vi "Omniax_mDrive_COM9.vi"() -> ()   [LabVIEW 2009]
uses:
  <vilib>/Instr/_visa.llb/VISA Configure Serial Port (Instr).vi
panel:
  out "Holding Current %":i32
  out "Run Current %":i32
  out "slew velocity mm/sec":dbl
  out "slew length mm":dbl
  in  "Slew Cancel":bool
  out "Position mm":dbl
  out "offset":dbl
  out "mm/rev":dbl
  out "step/rev":u32
  out "steps/sec":i32
  in  "Slew Length":i32 min=-80000 max=2000 step=100
  out "Slew Ready":bool
  in  "Slew Set":bool
  in  "Slew Go":bool
  in  "Velocity":i32 caption="steps/sec"
  in  "Slew Velocity":i32 min=1 max=1 step=1
  in  "Backlash":i32
  in  "Stop":bool
  out "In Range?":bool
  out "Current Values":i32 max=2000
  out "Status":string
  in  "Go":bool
  in  "Move to":i32=-20000 min=-80000 max=2000 step=500
  out "MINPOS":i32=-94296
  out "MAXPOS":i32=-34296
  out "COM PORT":refnum<visa-resource-name>="COM5"
  # "SY"
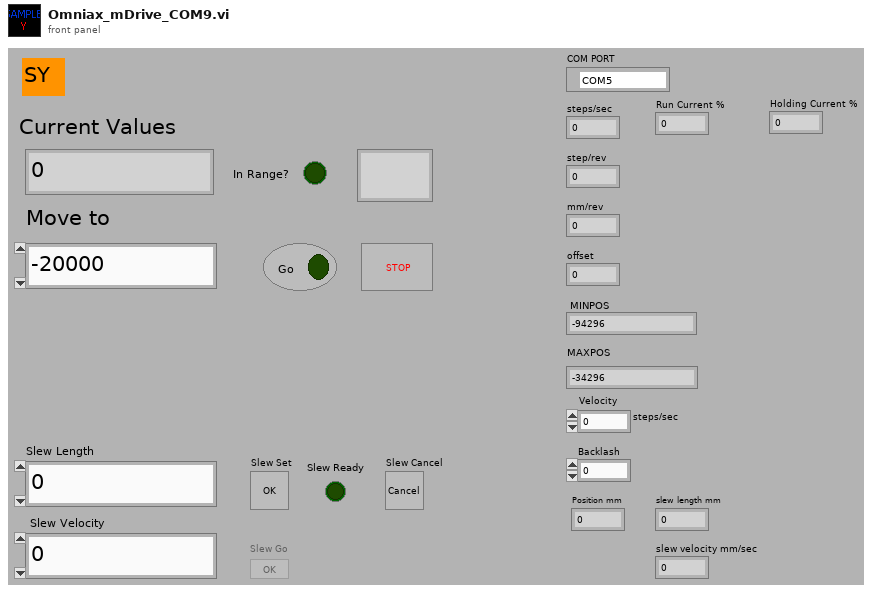
[diagram p1: front panel]
types:
  T1 = enum8{"Enabled", "Disabled", "Disabled and Grayed Out"}
  T2 = enum16{"Stop", "Reset", "Run Current", "Holding Current", "Accel Rate", "Decel Rate", "Move to Relative Position", "Move to Absolute Position", "Prtint Position", "Print Encorder", "Print Velocity Maximum", "Print Velocity", "Microstep Resolution", "Hold", "Max Velocity"}
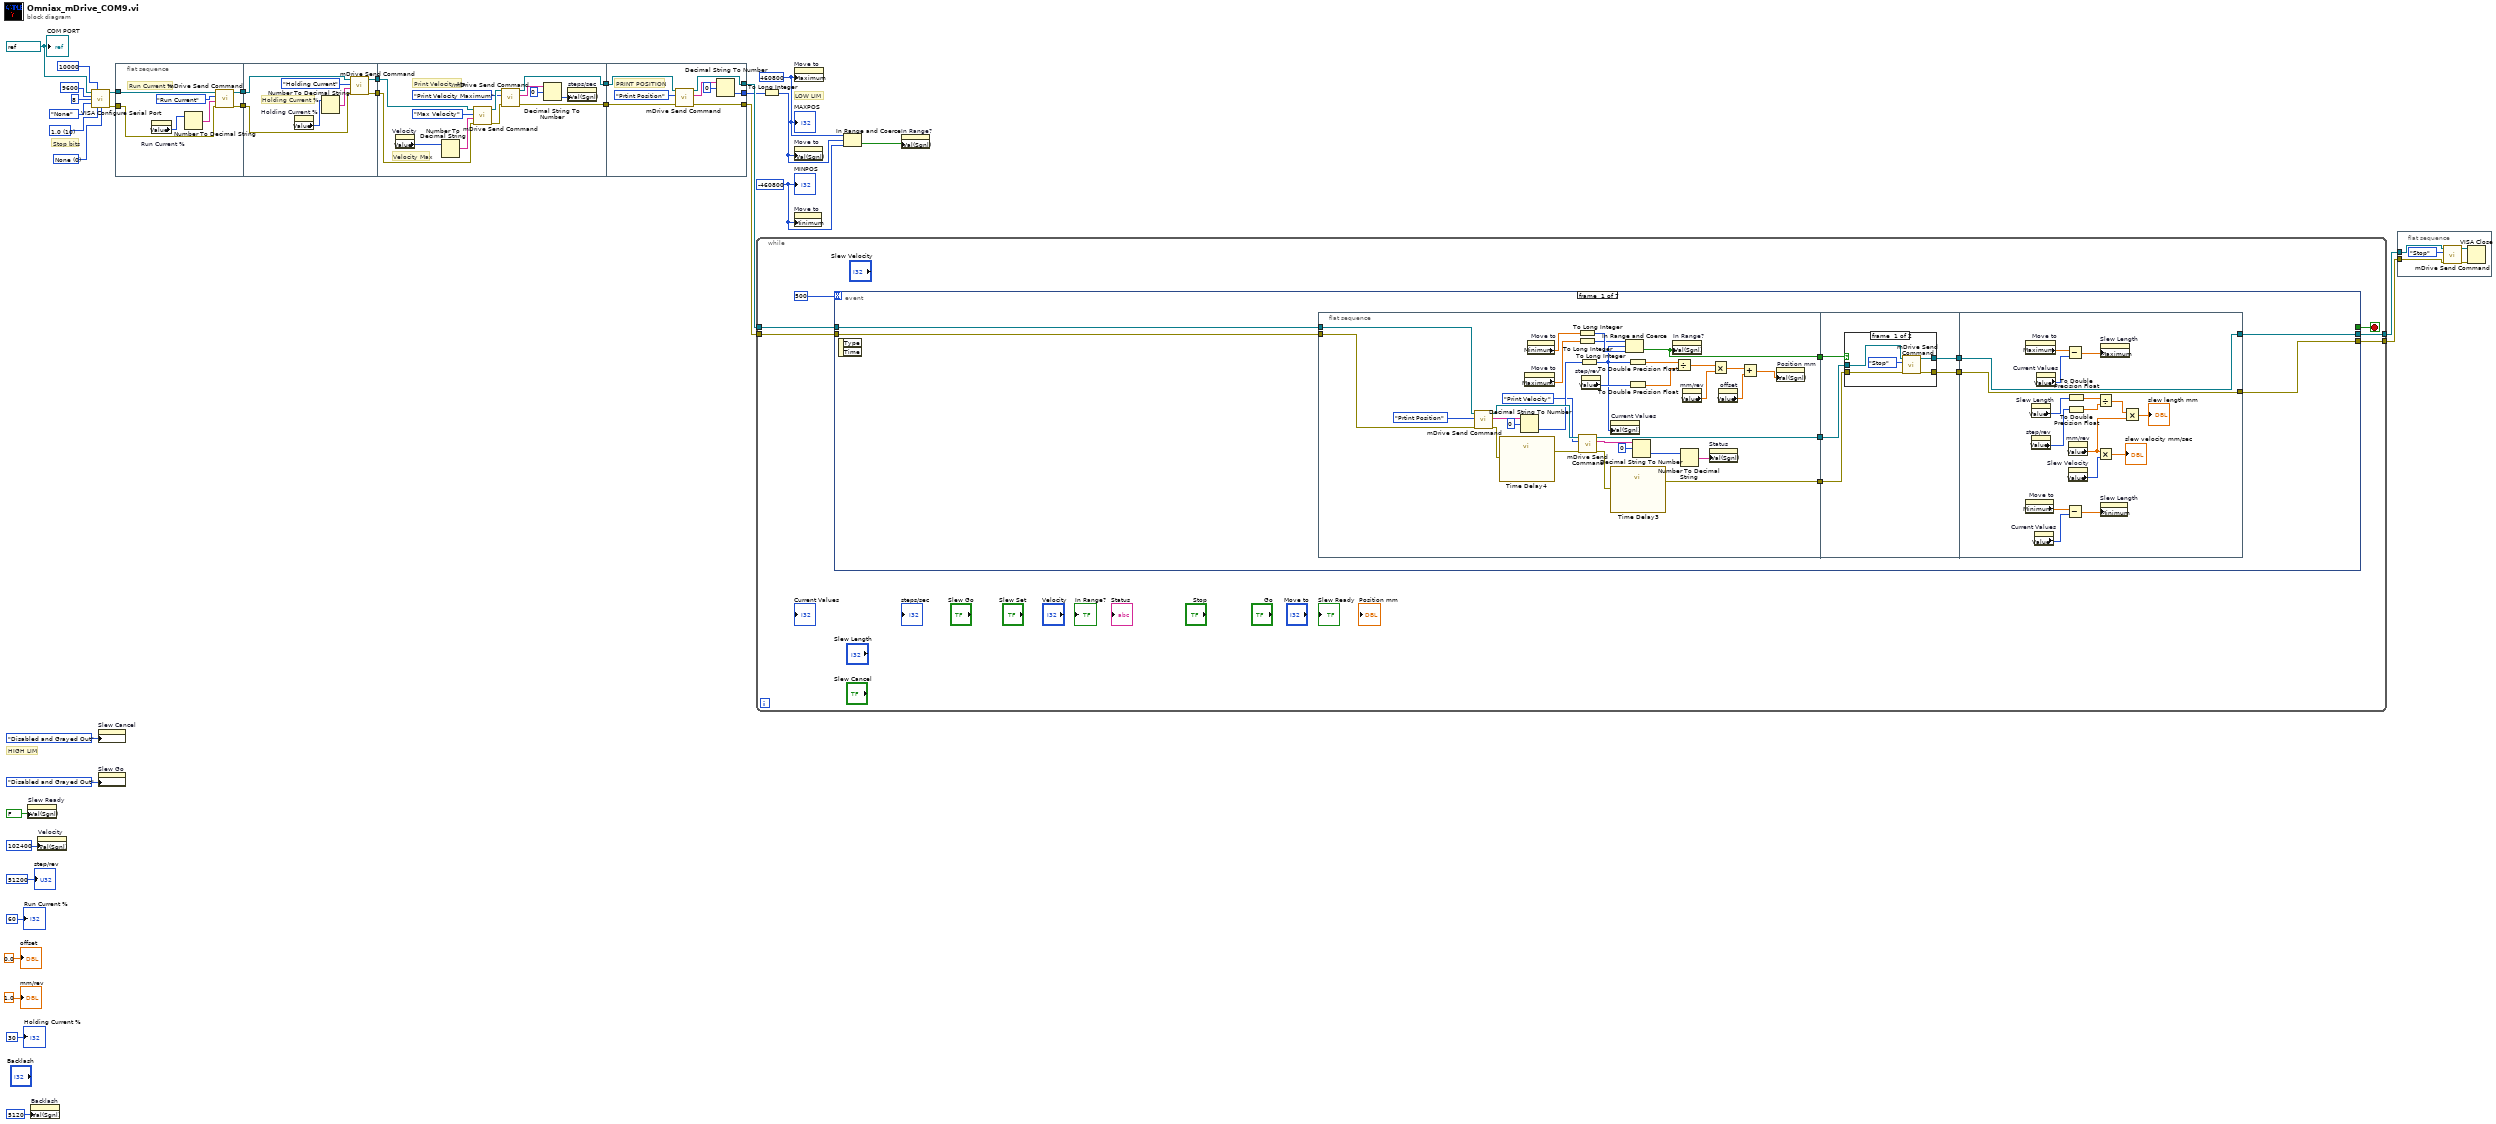
[diagram p0: block diagram]
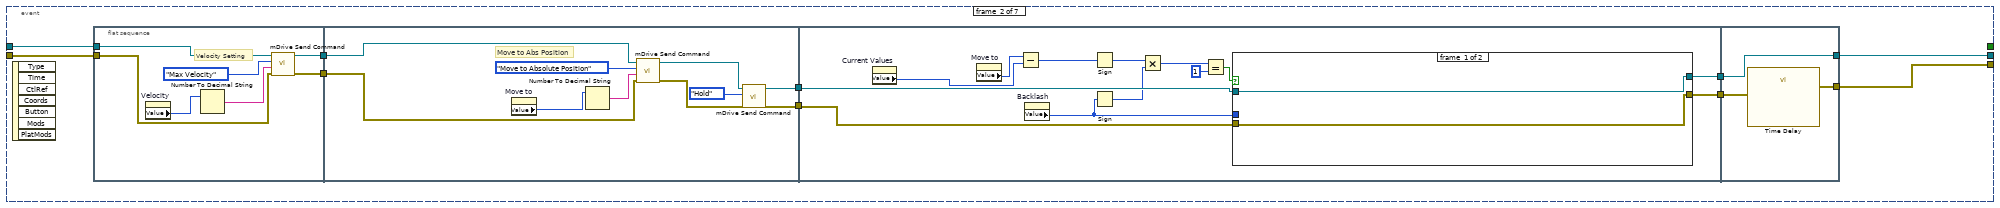
[diagram p3: hidden frame]
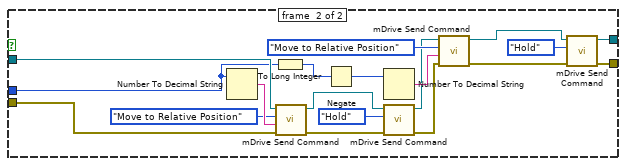
[diagram p4: hidden frame]
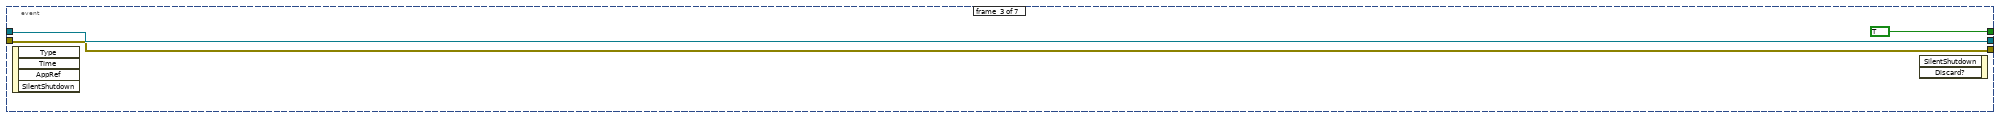
[diagram p5: hidden frame]
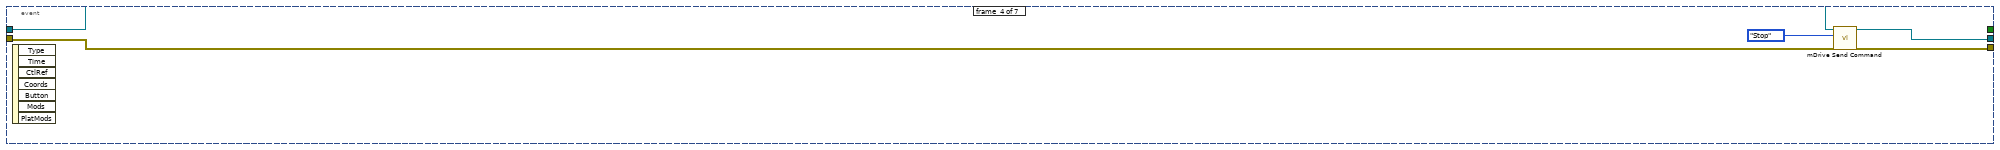
[diagram p6: hidden frame]
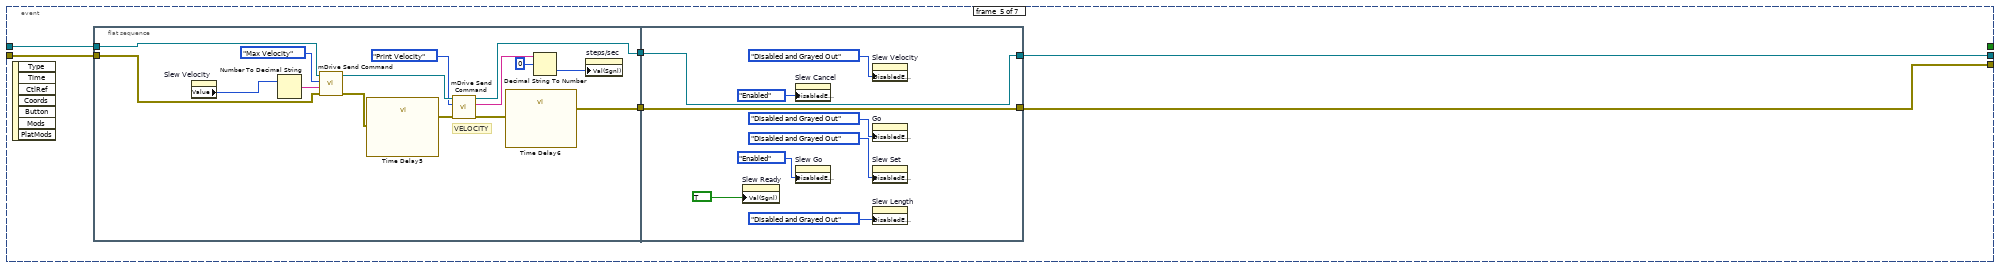
[diagram p7: hidden frame]
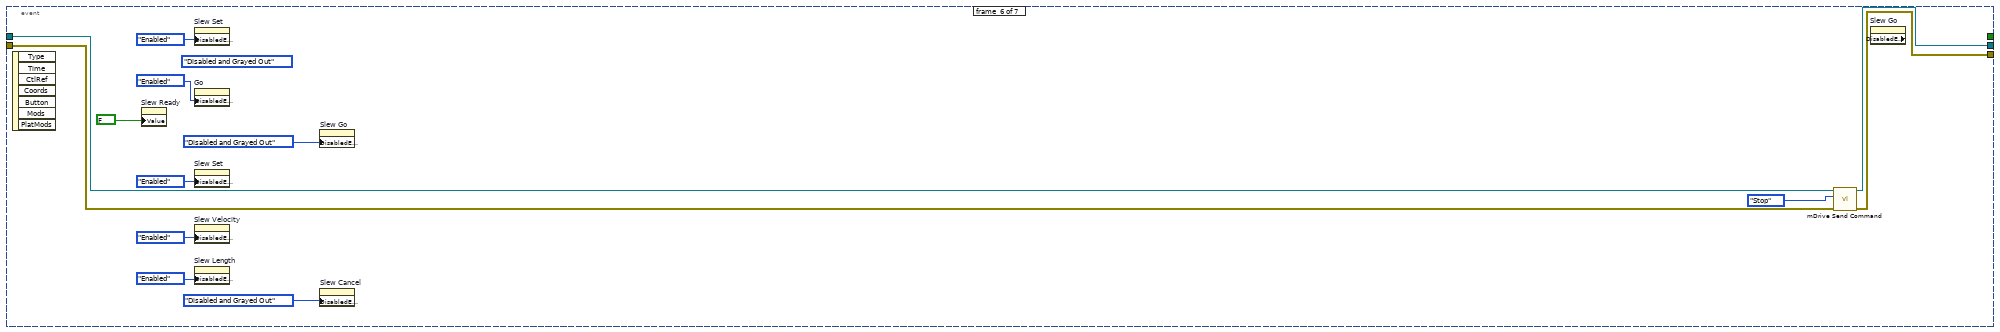
[diagram p8: hidden frame]
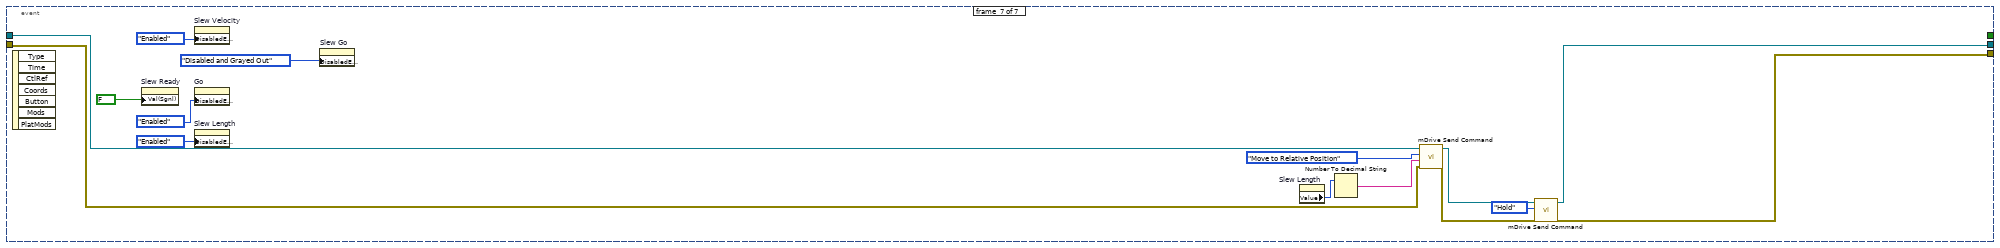
[diagram p9: hidden frame]
diagram:
  w20 = -460800 ("lower limit")
  w19 = 460800 ("upper limit")
  w28 = refnum<visa-resource-name> "COM9" ("COM PORT")
  w30 = u16 0 items=["None", "XON/XOFF", "RTS/CTS", "XON/XOFF & RTS/CTS", "DTR/DSR", "XON/XOFF & DTR/DSR"] ("flow control (0:none)")
  w31 = u16 10 items=["1.0"=10, "1.5"=15, "2.0"=20] ("stop bits (10: 1 bit)")
  # "HIGH LIM"
  # "LOW LIM"
  # "Stop bits"
  n1 = property on="Slew Ready" class="Bool (strict)"("Val(Sgnl)"=FALSE ("Value (Signaling)")) -> ()  [unwired: 2 in, 2 out]
  n2 = property on="Backlash" class="DigNum (strict)"("Val(Sgnl)"=u32 5120 ("Value (Signaling)")) -> ()  [unwired: 2 in, 2 out]
  n3 = property on="Velocity" class="DigNum (strict)"("Val(Sgnl)"=102400 ("Value (Signaling)")) -> ()  [unwired: 2 in, 2 out]
  n4 = call-poly "VISA Configure Serial Port"("VISA resource name"=w28, "timeout (10sec)"=u32 10000, "baud rate (9600)"=u32 9600, "data bits (8)"=u16 8, "parity (0:none)"=enum16{"None", "Odd", "Even", "Mark", "Space"}."None", "stop bits (10: 1 bit)"=w31, "flow control (0:none)"=w30) -> ("VISA resource name out"=w14:refnum<visa-resource-name>, "error out"=w13:errorcluster)  [unwired: 7 in]
  n5 = property on="Slew Cancel" class="Bool"("DisabledEnum"=T1."Disabled and Grayed Out" ("Disabled")) -> ()  [unwired: 2 in, 2 out]
  n6 = property on="Slew Go" class="Bool"("DisabledEnum"=T1."Disabled and Grayed Out" ("Disabled")) -> ()  [unwired: 2 in, 2 out]
  n7 = flat-sequence {
    tunnel: w13 -> [w41]
    tunnel: w14 -> [w39]
    tunnel: [w38] -> w6
    tunnel: [w40] -> w4
    tunnel: w6 -> [w48]
    tunnel: [w47] -> w5
    tunnel: w4 -> [w45]
    tunnel: [w46] -> w3
    tunnel: [w57] -> w16
    tunnel: [w58] -> w15
    tunnel: w5 -> [w56]
    tunnel: w3 -> [w55]
    tunnel: [w69] -> w27
    tunnel: [w68] -> w26
    tunnel: [w63] -> w17
    tunnel: w16 -> [w67]
    tunnel: w15 -> [w66]
    frame #0 {
      # "Run Current %"
      n8 = property on="Run Current %" class="DigNum (strict)"() -> ("Value"=w36:i32)  [unwired: 2 in, 2 out]
      n9 = Number To Decimal String(number=w36) -> (decimal integer string=w37:string)  [unwired: 1 in]
      n10 = call "mDrive Send Command.vi"("error in (no error)"=w41, "Extra"=w37, "Command"=T2."Run Current", "VISA resource name"=w39) -> ("error out"=w40:errorcluster, "VISA resource name out"=w38:refnum<visa-resource-name>)  [unwired: 3 in, 1 out]
    }
    frame #1 {
      # "Holding Current %"
      n11 = property on="Holding Current %" class="DigNum (strict)"() -> ("Value"=w43:i32)  [unwired: 2 in, 2 out]
      n12 = Number To Decimal String(number=w43) -> (decimal integer string=w44:string)  [unwired: 1 in]
      n13 = call "mDrive Send Command.vi"("error in (no error)"=w45, "Extra"=w44, "Command"=T2."Holding Current", "VISA resource name"=w48) -> ("error out"=w46:errorcluster, "VISA resource name out"=w47:refnum<visa-resource-name>)  [unwired: 3 in, 1 out]
    }
    frame #2 {
      # "Print Velocity Ma"
      # "Velocity Max"
      n14 = property on="Velocity" class="DigNum (strict)"() -> ("Value"=w54:i32)  [unwired: 2 in, 2 out]
      n15 = Number To Decimal String(number=w54) -> (decimal integer string=w53:string)  [unwired: 1 in]
      n16 = call "mDrive Send Command.vi"("error in (no error)"=w55, "Extra"=w53, "Command"=T2."Max Velocity", "VISA resource name"=w56) -> ("error out"=w51:errorcluster, "VISA resource name out"=w61:refnum<visa-resource-name>)  [unwired: 3 in, 1 out]
      n17 = call "mDrive Send Command.vi"("error in (no error)"=w51, "Command"=T2."Print Velocity Maximum", "VISA resource name"=w61) -> ("error out"=w58:errorcluster, "read buffer"=w59:string, "VISA resource name out"=w57:refnum<visa-resource-name>)  [unwired: 4 in]
      n18 = Decimal String To Number(string=w59, offset=0) -> (number=w52:i32)  [unwired: 1 in, 1 out]
      n19 = property on="steps/sec" class="DigNum (strict)"("Val(Sgnl)"=w52) -> ()  [unwired: 2 in, 2 out]
    }
    frame #3 {
      # "PRINT POSITION"
      n20 = call "mDrive Send Command.vi"("error in (no error)"=w66, "Command"=T2."Prtint Position", "VISA resource name"=w67) -> ("error out"=w68:errorcluster, "read buffer"=w65:string, "VISA resource name out"=w69:refnum<visa-resource-name>)  [unwired: 4 in]
      n21 = Decimal String To Number(string=w65, offset=0) -> (number=w63:i32)  [unwired: 1 in, 1 out]
    }
  }
  n22 = while {
    tunnel: w27 -> [w71]
    tunnel: w26 -> [w74]
    tunnel: [w75] -> w23
    tunnel: [w73] -> w24
    stop <- w70 stop-if-true
    n23 = event shown="[6] \"Slew Go\": Mouse Up" {
      selector: _ -> [_ _ _ _ _ _ _]
      dyn-events: _ -> [_ _ _ _ _ _ _]
      timeout: 500 -> [_ _ _ _ _ _ _]
      tunnel: w74 -> [w84 w154 w210 w215 w222 w252 w267]
      tunnel: [w83 w151 w210 w213 w220 w254 w261] -> w75
      tunnel: w71 -> [w81 w153 w211 w216 w221 w253 w266]
      tunnel: [w82 w152 w211 w214 w217 w255 w263] -> w73
      tunnel: [_ _ TRUE _ _ _ _] -> w70
      event #0 {
        n24 = event-data() -> ()  [unwired: 1 in, 2 out]
        n25 = flat-sequence {
          tunnel: w84 -> [w110]
          tunnel: w81 -> [w109]
          tunnel: [w115] -> w80
          tunnel: [w89] -> w78
          tunnel: [w102] -> w76
          tunnel: w80 -> [w117]
          tunnel: [w118] -> w79
          tunnel: w78 -> [w120]
          tunnel: [w119] -> w77
          tunnel: w76 -> [w116]
          tunnel: [w143] -> w83
          tunnel: [w144] -> w82
          tunnel: w79 -> [w144]
          tunnel: w77 -> [w143]
          frame #0 {
            n26 = call "mDrive Send Command.vi"("error in (no error)"=w110, "Command"=T2."Prtint Position", "VISA resource name"=w109) -> ("error out"=w108:errorcluster, "read buffer"=w114:string, "VISA resource name out"=w112:refnum<visa-resource-name>)  [unwired: 4 in]
            n27 = call "Time Delay4"("error in (no error)"=w108) -> ("error out"=w107:errorcluster)  [unwired: 10 in]
            n28 = Decimal String To Number(string=w114, offset=0) -> (number=w92:i32)  [unwired: 1 in, 1 out]
            n29 = property on="Move to" class="DigNum (strict)"() -> ("Maximum"=w104:dbl)  [unwired: 2 in, 2 out]
            n30 = property on="Move to" class="DigNum (strict)"() -> ("Minimum"=w106:dbl)  [unwired: 2 in, 2 out]
            n31 = To Long Integer(number=w106) -> (32bit integer=w105:i32)
            n32 = To Long Integer(number=w104) -> (32bit integer=w103:i32)
            n33 = call "mDrive Send Command.vi"("error in (no error)"=w107, "Command"=T2."Print Velocity", "VISA resource name"=w112) -> ("error out"=w111:errorcluster, "read buffer"=w90:string, "VISA resource name out"=w115:refnum<visa-resource-name>)  [unwired: 4 in]
            n34 = To Long Integer(number=w92) -> (32bit integer=w94:i32)
            n35 = property on="step/rev" class="DigNum (strict)"() -> ("Value"=w100:u32)  [unwired: 2 in, 2 out]
            n36 = property on="Current Values" class="DigNum (strict)"("Val(Sgnl)"=w94) -> ()  [unwired: 2 in, 2 out]
            n37 = call "Time Delay3"("error in (no error)"=w111) -> ("error out"=w89:errorcluster)  [unwired: 10 in]
            n38 = In Range and Coerce(upper limit=w103, x=w94, lower limit=w105) -> (In Range?=w102:bool)  [unwired: 1 out]
            n39 = To Double Precision Float(number=w94) -> (double precision float=w95:dbl)
            n40 = To Double Precision Float(number=w100) -> (double precision float=w101:dbl)
            n41 = Decimal String To Number(string=w90, offset=0 ("offset (0)")) -> (number=w88:i32)  [unwired: 1 in, 1 out]
            n42 = property on="In Range?" class="Bool (strict)"("Val(Sgnl)"=w102) -> ()  [unwired: 2 in, 2 out]
            n43 = Divide(x=w95, y=w101) -> (x/y=w99:dbl)
            n44 = Number To Decimal String(number=w88) -> (decimal integer string=w87:string)  [unwired: 1 in]
            n45 = property on="mm/rev" class="DigNum (strict)"() -> ("Value"=w98:dbl)  [unwired: 2 in, 2 out]
            n46 = property on="Status" class="Str"("Val(Sgnl)"=w87) -> ()  [unwired: 2 in, 2 out]
            n47 = Multiply(x=w99, y=w98) -> (x*y=w97:dbl)
            n48 = property on="offset" class="DigNum (strict)"() -> ("Value"=w96:dbl)  [unwired: 2 in, 2 out]
            n49 = Add(x=w97, y=w96) -> (x+y=w93:dbl)
            n50 = property on="Position mm" class="DigNum (strict)"("Val(Sgnl)"=w93) -> ()  [unwired: 2 in, 2 out]
          }
          frame #1 {
            n51 = case shown="False" w116 {
              tunnel: w117 -> [w123 w127]
              tunnel: [w124 w127] -> w118
              tunnel: [w125 w126] -> w119
              tunnel: w120 -> [w122 w126]
              frame #0 {
                n52 = call "mDrive Send Command.vi"("error in (no error)"=w122, "Command"=T2."Stop", "VISA resource name"=w123) -> ("error out"=w125:errorcluster, "VISA resource name out"=w124:refnum<visa-resource-name>)  [unwired: 4 in, 1 out]
              }
              frame #1 {
              }
            }
          }
          frame #2 {
            n53 = property on="Move to" class="DigNum (strict)"() -> ("Maximum"=w138:dbl)  [unwired: 2 in, 2 out]
            n54 = property on="Move to" class="DigNum (strict)"() -> ("Minimum"=w140:dbl)  [unwired: 2 in, 2 out]
            n55 = property on="Slew Length" class="DigNum (strict)"() -> ("Value"=w134:i32)  [unwired: 2 in, 2 out]
            n56 = property on="step/rev" class="DigNum (strict)"() -> ("Value"=w132:u32)  [unwired: 2 in, 2 out]
            n57 = property on="Current Values" class="DigNum (strict)"() -> ("Value"=w142:i32)  [unwired: 2 in, 2 out]
            n58 = property on="Current Values" class="DigNum (strict)"() -> ("Value"=w139:i32)  [unwired: 2 in, 2 out]
            n59 = Subtract(x=w138, y=w139) -> (x-y=w137:dbl)
            n60 = Subtract(x=w140, y=w142) -> (x-y=w141:dbl)
            n61 = To Double Precision Float(number=w134) -> (double precision float=w133:dbl)
            n62 = To Double Precision Float(number=w132) -> (double precision float=w136:dbl)
            n63 = property on="mm/rev" class="DigNum (strict)"() -> ("Value"=w128:dbl)  [unwired: 2 in, 2 out]
            n64 = property on="Slew Velocity" class="DigNum (strict)"() -> ("Value"=w130:i32)  [unwired: 2 in, 2 out]
            n65 = Divide(x=w133, y=w136) -> (x/y=w135:dbl)
            n66 = Multiply(x=w128, y=w130) -> (x*y=→"slew velocity mm/sec":dbl)
            n67 = property on="Slew Length" class="DigNum (strict)"("Maximum"=w137) -> ()  [unwired: 2 in, 2 out]
            n68 = property on="Slew Length" class="DigNum (strict)"("Minimum"=w141) -> ()  [unwired: 2 in, 2 out]
            n69 = Multiply(x=w135, y=w128) -> (x*y=→"slew length mm":dbl)
          }
        }
      }
      event #1 {
        n70 = event-data() -> ()  [unwired: 1 in, 7 out]
        n71 = flat-sequence {
          tunnel: w153 -> [w157]
          tunnel: w154 -> [w160]
          tunnel: [w159] -> w147
          tunnel: [w158] -> w146
          tunnel: w147 -> [w170]
          tunnel: w146 -> [w171]
          tunnel: [w165] -> w150
          tunnel: [w163] -> w148
          tunnel: w150 -> [w184]
          tunnel: [w181] -> w149
          tunnel: w148 -> [w183]
          tunnel: [w182] -> w145
          tunnel: [w207] -> w151
          tunnel: [w208] -> w152
          tunnel: w149 -> [w208]
          tunnel: w145 -> [w206]
          frame #0 {
            # "Velocity Setting"
            n72 = property on="Velocity" class="DigNum (strict)"() -> ("Value"=w161:i32)  [unwired: 2 in, 2 out]
            n73 = Number To Decimal String(number=w161) -> (decimal integer string=w156:string)  [unwired: 1 in]
            n74 = call "mDrive Send Command.vi"("error in (no error)"=w160, "Extra"=w156, "Command"=T2."Max Velocity", "VISA resource name"=w157) -> ("error out"=w159:errorcluster, "VISA resource name out"=w158:refnum<visa-resource-name>)  [unwired: 3 in, 1 out]
          }
          frame #1 {
            # "Move to Abs Position"
            n75 = property on="Move to" class="DigNum (strict)"() -> ("Value"=w169:i32)  [unwired: 2 in, 2 out]
            n76 = Number To Decimal String(number=w169) -> (decimal integer string=w168:string)  [unwired: 1 in]
            n77 = call "mDrive Send Command.vi"("error in (no error)"=w170, "Extra"=w168, "Command"=T2."Move to Absolute Position", "VISA resource name"=w171) -> ("error out"=w164:errorcluster, "VISA resource name out"=w166:refnum<visa-resource-name>)  [unwired: 3 in, 1 out]
            n78 = call "mDrive Send Command.vi"("error in (no error)"=w164, "Command"=T2."Hold", "VISA resource name"=w166) -> ("error out"=w163:errorcluster, "VISA resource name out"=w165:refnum<visa-resource-name>)  [unwired: 4 in, 1 out]
          }
          frame #2 {
            n79 = property on="Current Values" class="DigNum (strict)"() -> ("Value"=w179:i32)  [unwired: 2 in, 2 out]
            n80 = property on="Move to" class="DigNum (strict)"() -> ("Value"=w180:i32)  [unwired: 2 in, 2 out]
            n81 = Subtract(x=w180, y=w179) -> (x-y=w178:i32)
            n82 = property on="Backlash" class="DigNum (strict)"() -> ("Value"=w172:i32)  [unwired: 2 in, 2 out]
            n83 = Sign(1:w178) -> (0:w177:i32)
            n84 = Sign(1:w172) -> (0:w176:i32)
            n85 = Multiply(x=w177, y=w176) -> (x*y=w175:i32)
            n86 = Equal?(x=w175, y=1) -> (x = y?=w173:bool)
            n87 = case shown="True" w173 {
              tunnel: w184 -> [w186 w205]
              tunnel: [w186 w187] -> w181
              tunnel: [w185 w189] -> w182
              tunnel: w183 -> [w185 w204]
              tunnel: w172 -> [_ w199]
              frame #0 {
              }
              frame #1 {
                n88 = Number To Decimal String(number=w199) -> (decimal integer string=w203:string)  [unwired: 1 in]
                n89 = To Long Integer(number=w199) -> (32bit integer=w201:i32)
                n90 = call "mDrive Send Command.vi"("error in (no error)"=w204, "Extra"=w203, "Command"=T2."Move to Relative Position", "VISA resource name"=w205) -> ("error out"=w196:errorcluster, "VISA resource name out"=w194:refnum<visa-resource-name>)  [unwired: 3 in, 1 out]
                n91 = Negate(x=w201) -> (-x=w202:i32)
                n92 = Number To Decimal String(number=w202) -> (decimal integer string=w200:string)  [unwired: 1 in]
                n93 = call "mDrive Send Command.vi"("error in (no error)"=w196, "Command"=T2."Hold", "VISA resource name"=w194) -> ("error out"=w195:errorcluster, "VISA resource name out"=w193:refnum<visa-resource-name>)  [unwired: 4 in, 1 out]
                n94 = call "mDrive Send Command.vi"("error in (no error)"=w195, "Extra"=w200, "Command"=T2."Move to Relative Position", "VISA resource name"=w193) -> ("error out"=w190:errorcluster, "VISA resource name out"=w188:refnum<visa-resource-name>)  [unwired: 3 in, 1 out]
                n95 = call "mDrive Send Command.vi"("error in (no error)"=w190, "Command"=T2."Hold", "VISA resource name"=w188) -> ("error out"=w189:errorcluster, "VISA resource name out"=w187:refnum<visa-resource-name>)  [unwired: 4 in, 1 out]
              }
            }
          }
          frame #3 {
            n96 = call "Time Delay"("error in (no error)"=w206) -> ("error out"=w207:errorcluster)  [unwired: 10 in]
          }
        }
      }
      event #2 {
        n97 = event-data() -> ()  [unwired: 1 in, 4 out]
        n98 = event-data() -> ()  [unwired: 3 in, 1 out]
      }
      event #3 {
        n99 = event-data() -> ()  [unwired: 1 in, 7 out]
        n100 = call "mDrive Send Command.vi"("error in (no error)"=w215, "Command"=T2."Stop", "VISA resource name"=w216) -> ("error out"=w213:errorcluster, "VISA resource name out"=w214:refnum<visa-resource-name>)  [unwired: 4 in, 1 out]
      }
      event #4 {
        n101 = event-data() -> ()  [unwired: 1 in, 7 out]
        n102 = flat-sequence {
          tunnel: w222 -> [w231]
          tunnel: w221 -> [w230]
          tunnel: [w227] -> w219
          tunnel: [w225] -> w218
          tunnel: [w245] -> w220
          tunnel: [w246] -> w217
          tunnel: w219 -> [w246]
          tunnel: w218 -> [w245]
          frame #0 {
            # "VELOCITY"
            n103 = property on="Slew Velocity" class="DigNum (strict)"() -> ("Value"=w228:i32)  [unwired: 2 in, 2 out]
            n104 = Number To Decimal String(number=w228) -> (decimal integer string=w229:string)  [unwired: 1 in]
            n105 = call "mDrive Send Command.vi"("error in (no error)"=w231, "Extra"=w229, "Command"=T2."Max Velocity", "VISA resource name"=w230) -> ("error out"=w232:errorcluster, "VISA resource name out"=w237:refnum<visa-resource-name>)  [unwired: 3 in, 1 out]
            n106 = call "Time Delay5"("error in (no error)"=w232) -> ("error out"=w235:errorcluster)  [unwired: 10 in]
            n107 = call "mDrive Send Command.vi"("error in (no error)"=w235, "Command"=T2."Print Velocity", "VISA resource name"=w237) -> ("error out"=w226:errorcluster, "read buffer"=w233:string, "VISA resource name out"=w227:refnum<visa-resource-name>)  [unwired: 4 in]
            n108 = call "Time Delay6"("error in (no error)"=w226) -> ("error out"=w225:errorcluster)  [unwired: 10 in]
            n109 = Decimal String To Number(string=w233, offset=0) -> (number=w236:i32)  [unwired: 1 in, 1 out]
            n110 = property on="steps/sec" class="DigNum (strict)"("Val(Sgnl)"=w236) -> ()  [unwired: 2 in, 2 out]
          }
          frame #1 {
            n111 = property on="Slew Ready" class="Bool (strict)"("Val(Sgnl)"=TRUE ("Slew Ready 2")) -> ()  [unwired: 2 in, 2 out]
            n112 = property on="Slew Cancel" class="Bool"("DisabledEnum"=T1."Enabled" ("Disabled")) -> ()  [unwired: 2 in, 2 out]
            n113 = property on="Slew Go" class="Bool"("DisabledEnum"=T1."Enabled" ("Disabled")) -> ()  [unwired: 2 in, 2 out]
            n114 = property on="Slew Velocity" class="DigNum (strict)"("DisabledEnum"=T1."Disabled and Grayed Out" ("Disabled")) -> ()  [unwired: 2 in, 2 out]
            n115 = property on="Go" class="Bool"("DisabledEnum"=T1."Disabled and Grayed Out" ("Disabled")) -> ()  [unwired: 2 in, 2 out]
            n116 = property on="Slew Set" class="Bool"("DisabledEnum"=T1."Disabled and Grayed Out" ("Disabled")) -> ()  [unwired: 2 in, 2 out]
            n117 = property on="Slew Length" class="DigNum (strict)"("DisabledEnum"=T1."Disabled and Grayed Out" ("Disabled")) -> ()  [unwired: 2 in, 2 out]
          }
        }
      }
      event #5 {
        (unwired) T1."Disabled and Grayed Out" ("Disabled")
        n118 = event-data() -> ()  [unwired: 1 in, 7 out]
        n119 = property on="Slew Ready" class="Bool (strict)"("Value"=FALSE ("Slew Ready")) -> ()  [unwired: 2 in, 2 out]
        n120 = property on="Slew Set" class="Bool"("DisabledEnum"=T1."Enabled" ("Disabled")) -> ()  [unwired: 2 in, 2 out]
        n121 = property on="Go" class="Bool"("DisabledEnum"=T1."Enabled" ("Disabled")) -> ()  [unwired: 2 in, 2 out]
        n122 = property on="Slew Set" class="Bool"("DisabledEnum"=T1."Enabled" ("Disabled")) -> ()  [unwired: 2 in, 2 out]
        n123 = property on="Slew Velocity" class="DigNum (strict)"("DisabledEnum"=T1."Enabled" ("Disabled")) -> ()  [unwired: 2 in, 2 out]
        n124 = property on="Slew Length" class="DigNum (strict)"("DisabledEnum"=T1."Enabled" ("Disabled")) -> ()  [unwired: 2 in, 2 out]
        n125 = property on="Slew Go" class="Bool"("DisabledEnum"=T1."Disabled and Grayed Out" ("Disabled")) -> ()  [unwired: 2 in, 2 out]
        n126 = property on="Slew Cancel" class="Bool"("DisabledEnum"=T1."Disabled and Grayed Out" ("Disabled")) -> ()  [unwired: 2 in, 2 out]
        n127 = call "mDrive Send Command.vi"("error in (no error)"=w252, "Command"=T2."Stop", "VISA resource name"=w253) -> ("error out"=w254:errorcluster, "VISA resource name out"=w255:refnum<visa-resource-name>)  [unwired: 4 in, 1 out]
        n128 = property on="Slew Go" class="Bool" props=["DisabledEnum"]() -> ()  [unwired: 2 in, 3 out]
      }
      event #6 {
        n129 = event-data() -> ()  [unwired: 1 in, 7 out]
        n130 = property on="Slew Ready" class="Bool (strict)"("Val(Sgnl)"=FALSE ("Slew Ready 2")) -> ()  [unwired: 2 in, 2 out]
        n131 = property on="Slew Velocity" class="DigNum (strict)"("DisabledEnum"=T1."Enabled" ("Disabled")) -> ()  [unwired: 2 in, 2 out]
        n132 = property on="Go" class="Bool"("DisabledEnum"=T1."Enabled" ("Disabled")) -> ()  [unwired: 2 in, 2 out]
        n133 = property on="Slew Length" class="DigNum (strict)"("DisabledEnum"=T1."Enabled" ("Disabled")) -> ()  [unwired: 2 in, 2 out]
        n134 = property on="Slew Go" class="Bool"("DisabledEnum"=T1."Disabled and Grayed Out" ("Disabled")) -> ()  [unwired: 2 in, 2 out]
        n135 = property on="Slew Length" class="DigNum (strict)"() -> ("Value"=w268:i32)  [unwired: 2 in, 2 out]
        n136 = Number To Decimal String(number=w268) -> (decimal integer string=w274:string)  [unwired: 1 in]
        n137 = call "mDrive Send Command.vi"("error in (no error)"=w267, "Extra"=w274, "Command"=T2."Move to Relative Position", "VISA resource name"=w266) -> ("error out"=w262:errorcluster, "VISA resource name out"=w264:refnum<visa-resource-name>)  [unwired: 3 in, 1 out]
        n138 = call "mDrive Send Command.vi"("error in (no error)"=w262, "Command"=T2."Hold", "VISA resource name"=w264) -> ("error out"=w261:errorcluster, "VISA resource name out"=w263:refnum<visa-resource-name>)  [unwired: 4 in, 1 out]
      }
    }
  }
  n139 = To Long Integer(number=w17) -> (32bit integer=w25:i32)
  n140 = property on="Move to" class="DigNum (strict)"("Maximum"=w19) -> ()  [unwired: 2 in, 2 out]
  n141 = property on="Move to" class="DigNum (strict)"("Val(Sgnl)"=w25) -> ()  [unwired: 2 in, 2 out]
  n142 = property on="Move to" class="DigNum (strict)"("Minimum"=w20) -> ()  [unwired: 2 in, 2 out]
  n143 = In Range and Coerce(upper limit=w19, x=w25, lower limit=w20) -> (In Range?=w22:bool)  [unwired: 1 out]
  n144 = property on="In Range?" class="Bool (strict)"("Val(Sgnl)"=w22) -> ()  [unwired: 2 in, 2 out]
  n145 = flat-sequence {
    tunnel: w24 -> [w279]
    tunnel: w23 -> [w276]
    frame #0 {
      n146 = call "mDrive Send Command.vi"("error in (no error)"=w276, "Command"=T2."Stop", "VISA resource name"=w279) -> ("error out"=w277:errorcluster, "VISA resource name out"=w278:refnum<visa-resource-name>)  [unwired: 4 in, 1 out]
      n147 = VISA Close(VISA resource name=w278, error in (no error)=w277) -> ()  [unwired: 1 out]
    }
  }
  "COM PORT" <- w28
  "MINPOS" <- w20
  "MAXPOS" <- w19
  "step/rev" <- u32 51200 ("step/rev")
  "mm/rev" <- 1.0 ("MM/rev")
  "offset" <- 0.0 ("offset")
  "Run Current %" <- 60 ("Run Current %")
  "Holding Current %" <- 30 ("Holding Current %")
